vi "HG00.vi"() -> ()   [LabVIEW 2019]
panel:
  in  "Array 4":dbl[](array[numeric])
  in  "Array 2":dbl[](array[numeric])
  out "return value 2":dbl[](array[numeric])
  out "error out":errorcluster
  in  "Python version":string="3.6"
  in  "function name":string="modes_from_1d_array"
  in  "module path":path=path "C:/Users/edwar/OneDrive/Documents/GitHub/Python-HG-Modes/HG Modes/PauLisa.py"
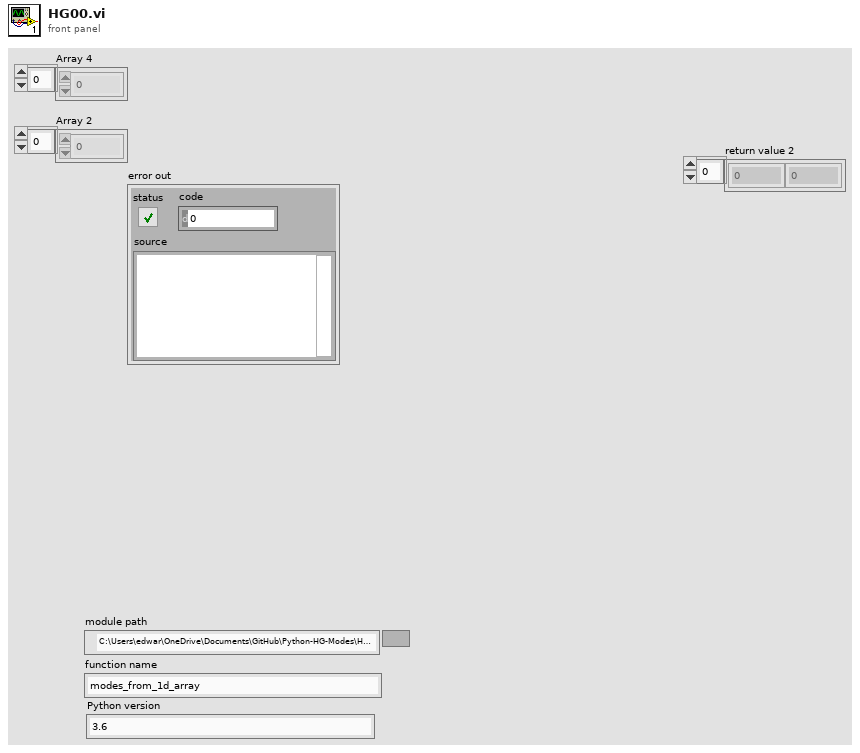
[diagram p1: front panel]
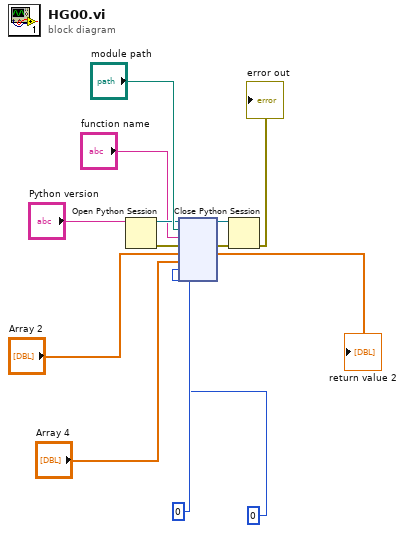
[diagram p0: block diagram]
diagram:
  n1 = Open Python Session(python version="Python version") -> (session out=w11:refnum<k35>, error out=w8:errorcluster)  [unwired: 2 in]
  n2 = node(w11, "module path", "function name", w8, "Array 2", "Array 4", 0, 0) -> (w10:refnum<k35>, w7:errorcluster, →"return value 2":dbl[])  [unwired: 3 in, 2 out]
  "error out" <- w7
  n3 = Close Python Session(session in=w10, error in=w7) -> ()  [unwired: 1 out]
